vi "XIPIN_Virtex-5_FPGA_RocketIO_GTP_Transceiver_Wizard_2_1.vi"   [LabVIEW 2017]
doc: "Use the Virtex-5 FPGA RocketIO GTP Transceiver Wizard to configure one or more Virtex-5 FPGA GTP transceivers. Start from scratch, or use an industry standard template. The Wizard generates a custom wrapper for the tranceivers you've selected. In addition, it produces an example design, testbench, and scripts to observe the transceivers operating under simulation and in hardware.\n------------------------------------\n<b>Need License</b> : No"
uses:
  <vilib>/rvi/XilinxIP/XIPIN_XNode/niFpgaXIPIN.xnode
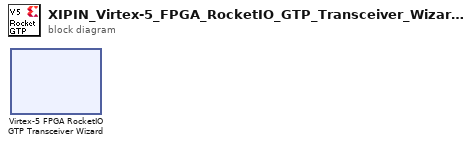
[diagram p0: block diagram]
diagram:
  n1 = xnode ("Virtex-5 FPGA RocketIO GTP Transceiver Wizard")() -> ()
